vi "XDataNode10_0To9_0.vi"(10 "Version-State Cluster In":T1, 11 "XRef":refnum<vi>) -> (0 "Custom Label":string, 1 "Custom Warning To Issue":string, 2 "Version-State Cluster Out":T1, 3 "Action":T2)   [LabVIEW 2017]
uses:
  <vilib>/XSFPSupport/SFPChangeStateAction.ctl
  <vilib>/XNodeSupport/XNodeVersion.ctl
  <vilib>/XNodeSupport/XNodeUShort.ctl
  <vilib>/Platform/TimedLoop/XDataNode/XDataNode.ctl
  <vilib>/Platform/TimedLoop/XDataNode/timing_clust.ctl
  <vilib>/Platform/TimedLoop/XDataNode/nitl_modes.ctl
  <vilib>/Platform/TimedLoop/XDataNode/wakeup.ctl
  <vilib>/Platform/TimedLoop/XDataNode/TermInfo.ctl
  <vilib>/Platform/TimedLoop/XDataNode/nitl_TargetSpecificData.ctl
  <vilib>/Platform/TimedLoop/XDataNode/DN_Type.ctl
  <vilib>/XSFPSupport/NI_XSFPSupport.lvlib
  <vilib>/XNodeSupport/NI_XNodeSupport.lvlib
  <vilib>/Platform/TimedLoop/XDataNode/XDataNode.xnode
  <vilib>/Platform/TimedLoop/XDataNode/XDNodeRunTimeDep.lvlib
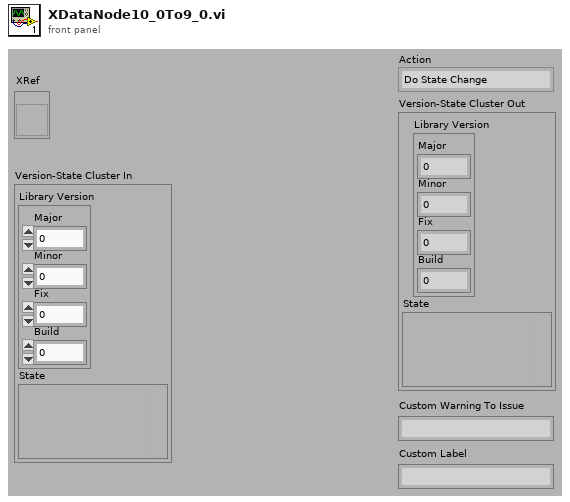
[diagram p1: front panel]
types:
  T1 = cluster{"Library Version":cluster{"Major":u16, "Minor":u16, "Fix":u16, "Build":u16}, "State":variant}
  T2 = typedef "NI_XSFPSupport.lvlib/SFPChangeStateAction.ctl" = enum32{"Do State Change", "Replace With Label", "Fail SFP"}
  T3 = typedef "XDataNode.xnode/XDataNode.ctl" = cluster{"Timing":T4, "Size":T7[], "Hidden":T7[], "Invisible":bool[], "Input?":bool, "timing src wired?":bool, "Target Specific Data":T8[], "G Only Data":variant, "DataNode_Type":T9}
  T4 = typedef "XDNodeRunTimeDep.lvlib/timing_clust.ctl" = cluster{"Expected End [f-1]":u64, "Actual End [f-1]":u64, "Finished Late? [f-1]":bool, "Expected End [i-1]":u64, "Actual End [i-1]":u64, "Finished Late? [i-1]":bool, "Expected Start [i]":u64, "Actual Start [i]":u64, "Expected Start [f]":u64, "Actual Start [f]":u64, "Source Name":string, "Structure Name":string, "Period":i64, "Deadline":i64, "Offset":i64, "Start":i64, "Priority":i32, "Timeout":i32, "Mode":T5, "Wakeup Reason":T6, "Error":errorcluster, "Source Type":string, "Secondary Source Type":string, "Global End Time":u64, "Global Start Time":u64, "Frame Duration":u64, "Iteration Duration":u64, "Assigned CPU":i32, "I/O Scan Engine Mode":u32}
  T5 = typedef "XDNodeRunTimeDep.lvlib/nitl_modes.ctl" = enum32{"No Change", "Process missed periods, maintain original phase", "Discard missed periods, maintain original phase", "Process missed periods, ignore original phase", "Discard missed periods, ignore original phase"}
  T6 = typedef "XDNodeRunTimeDep.lvlib/wakeup.ctl" = enum32{"Normal", "Aborted", "Asynchronous wakeup", "Timing source error", "Timed loop error", "Timeout"}
  T7 = typedef "XDataNode.xnode/TermInfo.ctl" = cluster{"ID":i32, "Wired?":bool, "Type":variant, "Name":string, "Input?":bool, "StaticID":i32}
  T8 = typedef "XDataNode.xnode/nitl_TargetSpecificData.ctl" = cluster{"Target Name":string, "Target Data":variant}
  T9 = typedef "XDataNode.xnode/DN_Type.ctl" = enum32{"TL_Lft_Ear", "TL_Rt_Ear", "TL_Lft_Dn", "TL_Rt_Dn", "TS_Lft_Ear", "TS_Rt_Ear", "TS_1stFrame_Lft_Dn", "TS_Lft_Dn", "TS_LastFrame_Rt_Dn", "TS_Rt_Dn", "TL_TS_Lft_Ear", "TL_TS_Rt_Ear", "TL_TS_Lft_Dn", "TL_TS_Rt_Dn", "TL_TS_1stFrame_Lft_Dn", "TL_TS_LastFrame_Rt_Dn"}
  T10 = typedef "NI_XNodeSupport.lvlib/XNodeVersion.ctl" = cluster{"Major":T11, "Minor":T11, "Fix":T11, "Build":T11}
  T11 = typedef "NI_XNodeSupport.lvlib/XNodeUShort.ctl" = u16
  T12 = cluster{"Major":u16, "Minor":u16, "Fix":u16, "Build":u16}
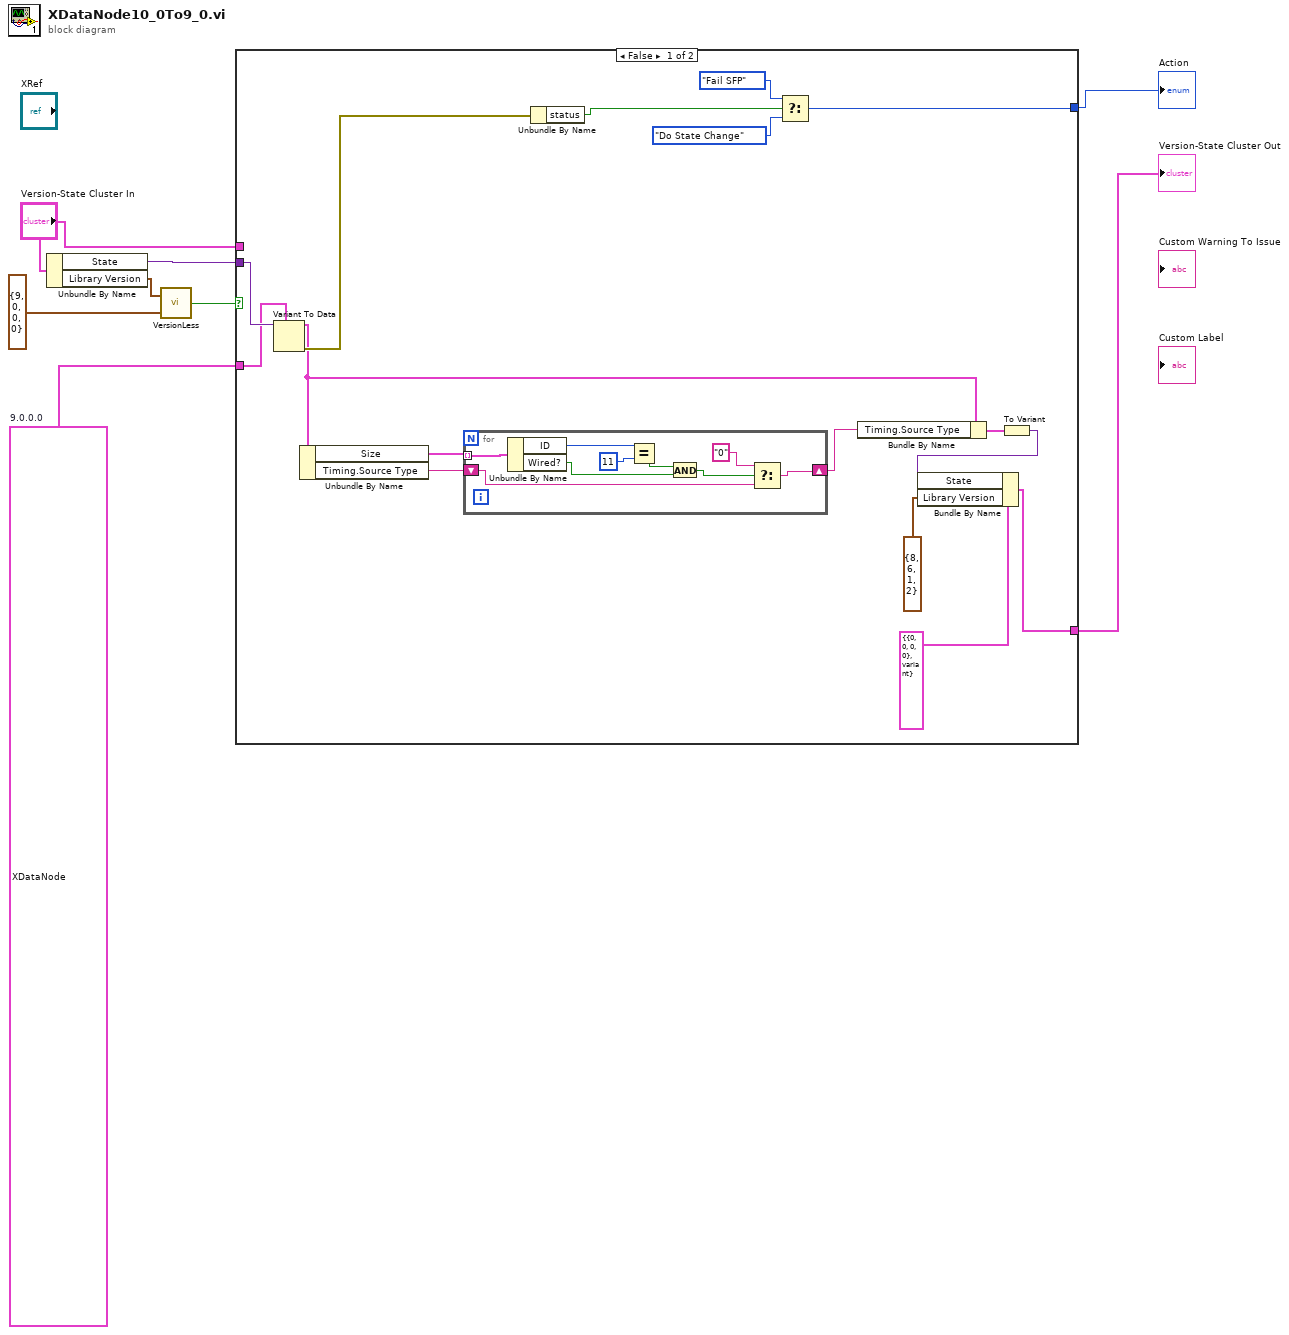
[diagram p0: block diagram]
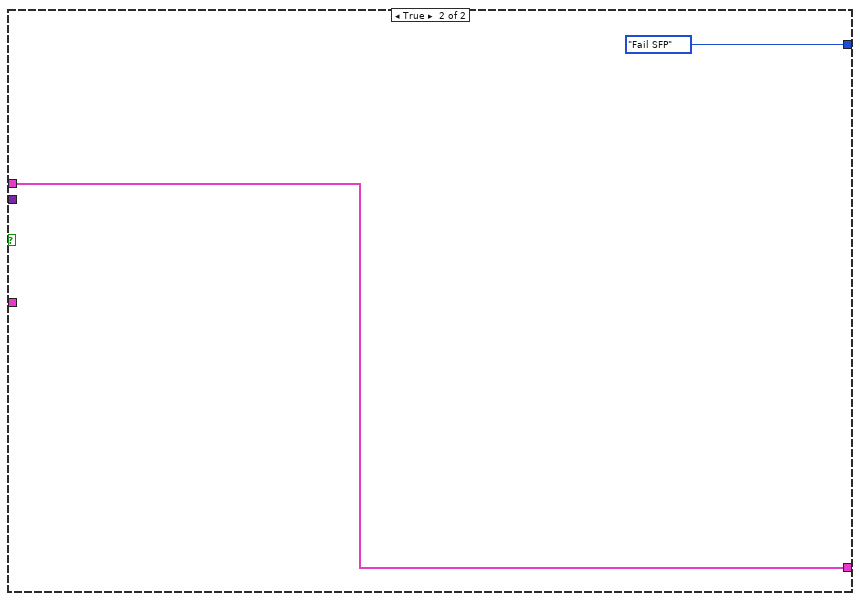
[diagram p2: hidden frame]
diagram:
  w3 = T3 {"Timing"={"Expected End [f-1]"=0, "Actual End [f-1]"=0, "Finished Late? [f-1]"=FALSE, "Expected End [i-1]"=0, "Actual End [i-1]"=0, "Finished Late? [i-1]"=FALSE, "Expected Start [i]"=0, "Actual Start [i]"=0, "Expected Start [f]"=0, "Actual Start [f]"=0, "Source Name"="", "Structure Name"="", "Period"=0, "Deadline"=0, "Offset"=0, "Start"=0, "Priority"=0, "Timeout"=0, "Mode"=enum."No Change", "Wakeup Reason"=enum."Normal", "Error"={"status"=FALSE, "code"=0, "source"=""}, "Source Type"="", "Secondary Source Type"="", "Global End Time"=0, "Global Start Time"=0, "Frame Duration"=0, "Iteration Duration"=0, "Assigned CPU"=0, "I/O Scan Engine Mode"=0}, "Size"=[], "Hidden"=[], "Invisible"=[], "Input?"=FALSE, "timing src wired?"=FALSE, "Target Specific Data"=[], "G Only Data"=variant, "DataNode_Type"=enum."TL_Lft_Ear"}  # 9.0.0.0
  n1 = Unbundle By Name("Version-State Cluster In") -> ("State"=w4:variant, "Library Version"=w5:T12)
  n2 = call <vilib>:"VersionLess.vi"("y"=T10 {"Major"=9, "Minor"=0, "Fix"=0, "Build"=0}, "x"=w5) -> ("x < y?"=w7:bool)
  n3 = case shown="False" w7 {
    tunnel: [w18 SFPChangeStateAction."Fail SFP" ("Action")] -> w6
    tunnel: w4 -> [w24 _]
    tunnel: w3 -> [w23 _]
    tunnel: [w13 w34] -> w2
    tunnel: "Version-State Cluster In" -> [_ w34]
    frame False {
      n4 = Variant To Data(type=w23, Variant=w24) -> (data=w12:T3, error out=w22:errorcluster)  [unwired: 1 in]
      n5 = Unbundle By Name(w12) -> ("Size"=w11:T7[], "Timing.Source Type"=w10:string)
      n6 = for {
        tunnel: w11 -> [w33] mode=indexing
        shift-right: [w27] -> w9
        shift-left: w10 -> [w26]
        n7 = Unbundle By Name(w33) -> ("ID"=w31:i32, "Wired?"=w29:bool)
        n8 = Equal?(x=w31, y=11) -> (x = y?=w30:bool)
        n9 = And(x=w30, y=w29) -> (x .and. y?=w28:bool)
        n10 = Select(t="0", s=w28, f=w26) -> (s? t:f=w27:string)
      }
      n11 = Unbundle By Name(w22) -> ("status"=w21:bool)
      n12 = Select(t=SFPChangeStateAction."Fail SFP" ("Action"), s=w21, f=SFPChangeStateAction."Do State Change" ("Action")) -> (s? t:f=w18:T2)
      n13 = Bundle By Name(cluster=w12, "Timing.Source Type"=w9) -> (w17:T3)
      n14 = To Variant(anything=w17) -> (Variant=w14:variant)
      n15 = Bundle By Name(cluster=T1 {"Library Version"={"Major"=0, "Minor"=0, "Fix"=0, "Build"=0}, "State"=variant} ("Version-State Cluster Out"), "State"=w14, "Library Version"=T10 {"Major"=8, "Minor"=6, "Fix"=1, "Build"=2} ("y")) -> (w13:T1)
    }
    frame True {
    }
  }
  "Action" <- w6
  "Version-State Cluster Out" <- w2
